vi "logic (core).vi"(8 "error in":errorcluster) -> (0 "error out":errorcluster, 2 "actual result":string)   [LabVIEW 2020, in "AIM ARINC 664 Import.lvclass"]
uses:
  AIM ARINC 664 Import.lvclass
  AIM ARINC 664 Import.lvclass/AIM ARINC 664 Import.ctl
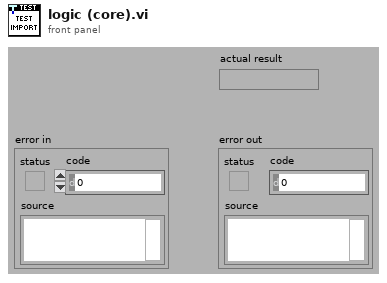
[diagram p1: front panel]
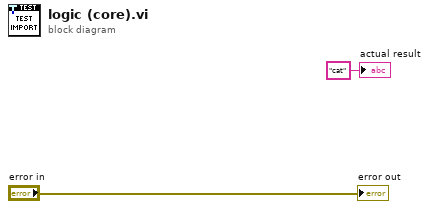
[diagram p0: block diagram]
diagram:
  "error out" <- "error in"
  "actual result" <- "cat" ("actual result")
